vi "Synchronize.vi"(11 "State":enum16{"Init", "Get"}(ring)=enum."Get") -> (3 "occurrence":refnum<k4>)   [LabVIEW 2014, in "Controller.lvlib" / "Controller.lvclass"]
uses:
  Controller.lvclass
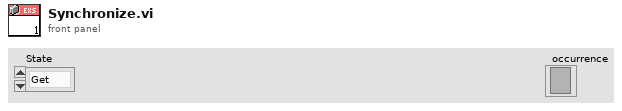
[diagram p1: front panel]
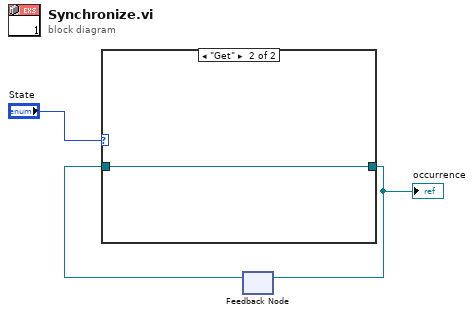
[diagram p0: block diagram]
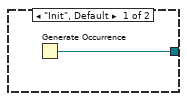
[diagram p2: hidden frame]
diagram:
  n1 = feedback #1() -> (w1:refnum<k4>)  [unwired: 1 in]
  n2 = case shown="\"Get\"" "State" {
    tunnel: [w4 w5] -> w2
    tunnel: w1 -> [_ w5]
    frame "Init", Default {
      n3 = Generate Occurrence() -> (w4:refnum<k4>)
    }
    frame "Get" {
    }
  }
  "occurrence" <- w2
  n4 = feedback-in #1(w2) -> ()
